vi "sub_NoiseEst_And_Chop_Shell.vi"(1 "data":cluster{"t0":dbl, "dt":dbl, "Y":cdb[]}, 3 "Enable":bool) -> (5 "Singal & Noise Power":cluster{"signal_power":dbl, "noise_power":dbl}, 6 "Output Packets":cluster{"Packets":cdb[][], "Enable?":bool}, 7 "Delay signal (for plotting use only)":cdb[](array[numeric]))   [LabVIEW 2015]
uses:
  sub_Ave_Power_And_Thresholding.vi
  sub_Extract_Packet_Boundaries - G.vi
  sub_Extract_Packets.vi
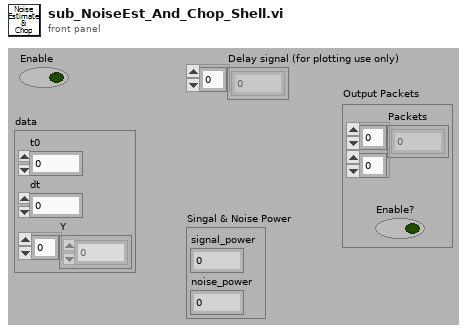
[diagram p1: front panel]
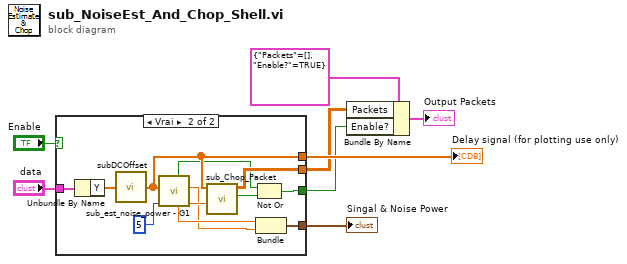
[diagram p0: block diagram]
diagram:
  n1 = case shown="Vrai" "Enable" {
    selector: "Enable" -> [w9 _]
    tunnel: "data" -> [_ w20]
    tunnel: [w9 w10] -> w3
    tunnel: [_ w18] -> w4
    tunnel: [_ w13] -> w7
    tunnel: [_ w17] -> w8
    frame False {
    }
    frame True {
      n2 = Unbundle By Name(w20) -> ("Y"=w14:cdb[])
      n3 = call "subDCOffset.vi"("Input signal samples"=w14) -> ("Output signal samples"=w13:cdb[])
      n4 = call "sub_est_noise_power - G1.vi"("Bin Size"=5, "Input Complex Samples"=w13) -> ("Energy Threshold"=w19:dbl, "noise_power"=w15:dbl, "signal_power"=w16:dbl, "noise_estimation_error ?"=w12:bool)  [unwired: 6 in]
      n5 = call "sub_Chop_Packet.vi"("Energy Threshold"=w19, "Input Complex Samples"=w13) -> ("Packet Detection Error?"=w11:bool, "packet_arr"=w18:cdb[][])  [unwired: 8 in]
      n6 = Not Or(1:w11, 2:w12) -> (0:w10:bool)
      n7 = Bundle("signal_power"=w16, "noise_power"=w15) -> (w17:cluster{"signal_power":dbl, "noise_power":dbl})  [unwired: 1 in]
    }
  }
  "Singal & Noise Power" <- w8
  "Delay signal (for plotting use only)" <- w7
  n8 = Bundle By Name(cluster=cluster{"Packets":cdb[][], "Enable?":bool} {"Packets"=[], "Enable?"=TRUE} ("Output Packets"), "Packets"=w4, "Enable?"=w3) -> (→"Output Packets":cluster{"Packets":cdb[][], "Enable?":bool})
